vi "DigitalInput.vi"(8 "discrete input values IN":bool[](array[boolean]), 11 "Digital Input Channel":T1(ring)) -> (0 "discrete input values OUT":bool[](array[boolean]), 3 "Digital Value":bool)   [LabVIEW 2025]
panel:
  # "Read single digital input from array\n\nReturns boolean value of desired phys. \npanel digital input. Stackable, wire in series\nor parallel for multiple contact reading.\n\nINPUTS:\n  1. Digital input channel -- int 0-7 or auto\n      configured enum DI-0 -> DI-7\n   2. Array of contactor values read from MB server.\n       boolean array with dimension 8x1\n\nOUTPUTS:\n   1. Value from channel selected with input 1.\n       Bool\n   2. Array of contactor values read from MB server.\n       boolean array with dimension 8x1 -- \n       Direct passthrough of input 2"
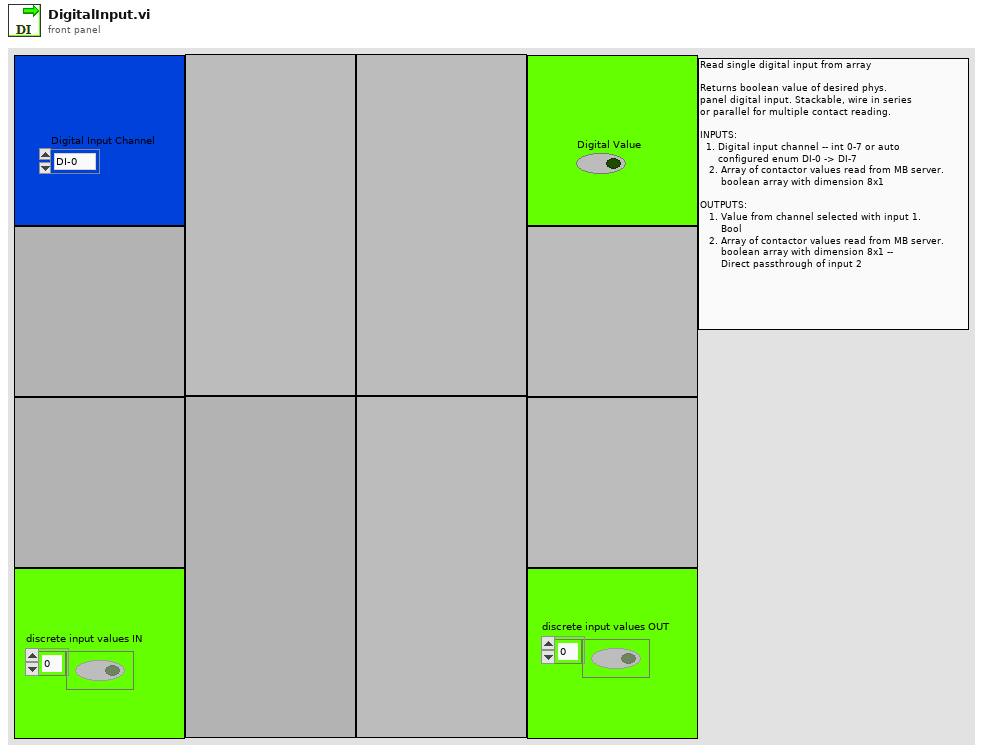
[diagram p1: front panel]
types:
  T1 = enum16{"DI-0", "DI-1", "DI-2", "DI-3", "DI-4", "DI-5", "DI-6", "DI-7"}
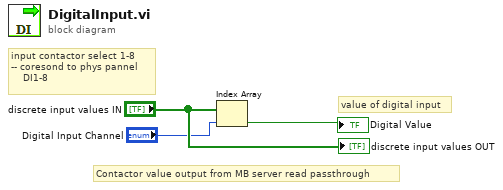
[diagram p0: block diagram]
diagram:
  # "value of digital input"
  # "Contactor value output from MB server read passthrough"
  # "input contactor select 1-8\n-- coresond to phys pannel\n    DI1-8"
  n1 = Index Array(array="discrete input values IN", index="Digital Input Channel") -> (element=→"Digital Value":bool)
  "discrete input values OUT" <- "discrete input values IN"
